vi "Tosca-Create Editor Event Registration.vi"(0 "FSM.Editor Ref":refnum<vi>, 5 "EventList Ref":refnum<vi>, 7 "Flags Ref":refnum<vi>, 9 "SigMan Ref":refnum<vi>) -> (4 "Event Registration Refnum":refnum<event-registration>)   [LabVIEW 2020]
uses:
  epl-vi-lib/Utility VIs/Controls/KListboxEx/KListboxEx.xctl
  FSM Graph VIs/LV Source/FSM Editor/FSM Editor.xctl
  epl-vi-lib/Utility VIs/Controls/KListboxEx/Events.ctl
  epl-vi-lib/Utility VIs/Controls/KListboxEx/Event Action.ctl
  epl-vi-lib/Utility VIs/Controls/KTable/KTable.xctl
  epl-vi-lib/Utility VIs/Controls/KTable/Events.ctl
  epl-vi-lib/Utility VIs/Controls/KTable/Event Data.ctl
  epl-vi-lib/Utility VIs/Controls/KTable/Event Type.ctl
  FSM Graph VIs/LV Source/FSM Editor/Events.ctl
  FSM Graph VIs/LV Source/FSM Editor/NodeAdded.ctl
  FSM Graph VIs/LV Source/FSM Editor/NodeSelected.ctl
  FSM Graph VIs/LV Source/FSM Editor/EdgeEventData.ctl
  epl-vi-lib/Signal Synthesis VIs/4th Generation/Controls/SignalManager/SignalManager.xctl
  epl-vi-lib/Signal Synthesis VIs/4th Generation/Controls/SignalManager/Events.ctl
  epl-vi-lib/Signal Synthesis VIs/4th Generation/Controls/SignalManager/Event Data.ctl
panel:
  out "SigMan":T1
  out "FSMEditor":T2
  out "Flags":T3
  out "EventList":T4
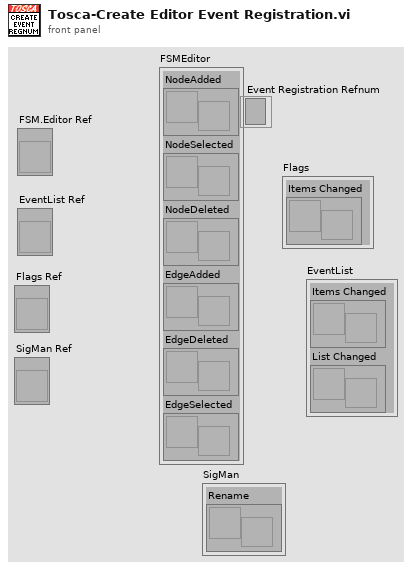
[diagram p1: front panel]
types:
  T1 = typedef "SignalManager.xctl/Events.ctl" = cluster{"Rename":refnum<user-event>}
  T2 = typedef "FSM Editor.xctl/Events.ctl" = cluster{"NodeAdded":refnum<user-event>, "NodeSelected":refnum<user-event>, "NodeDeleted":refnum<user-event>, "EdgeAdded":refnum<user-event>, "EdgeDeleted":refnum<user-event>, "EdgeSelected":refnum<user-event>}
  T3 = typedef "KTable.xctl/Events.ctl" = cluster{"Items Changed":refnum<user-event>}
  T4 = typedef "KListboxEx.xctl/Events.ctl" = cluster{"Items Changed":refnum<user-event>, "List Changed":refnum<user-event>}
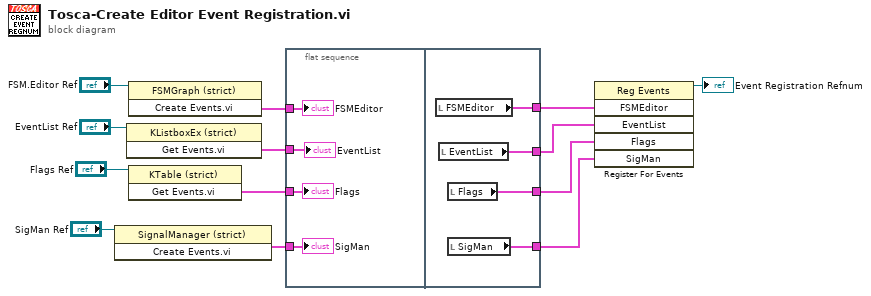
[diagram p0: block diagram]
diagram:
  n1 = invoke class="SignalManager (strict)" method="Create Events.vi"(reference="SigMan Ref") -> ("Create Events.vi"=w3:T1)  [unwired: 2 in, 2 out]
  n2 = invoke on="Invoke Node" class="KListboxEx (strict)" method="Get Events.vi"(reference="EventList Ref") -> ("Get Events.vi"=w10:T4)  [unwired: 2 in, 2 out]
  n3 = invoke on="Invoke Node" class="FSMGraph (strict)" method="Create Events.vi"(reference="FSM.Editor Ref") -> ("Create Events.vi"=w11:T2)  [unwired: 2 in, 2 out]
  n4 = invoke on="Invoke Node" class="KTable (strict)" method="Get Events.vi"(reference="Flags Ref") -> ("Get Events.vi"=w6:T3)  [unwired: 2 in, 2 out]
  n5 = flat-sequence {
    tunnel: w11 -> [w15]
    tunnel: w10 -> [w17]
    tunnel: w6 -> [w16]
    tunnel: w3 -> [w14]
    tunnel: [w21] -> w9
    tunnel: [w20] -> w8
    tunnel: [w19] -> w7
    tunnel: [w18] -> w2
    frame #0 {
      "EventList" <- w17
      "Flags" <- w16
      "FSMEditor" <- w15
      "SigMan" <- w14
    }
    frame #1 {
      n6 = local read "FSMEditor"() -> (w21:T2)
      n7 = local read "EventList"() -> (w20:T4)
      n8 = local read "Flags"() -> (w19:T3)
      n9 = local read "SigMan"() -> (w18:T1)
    }
  }
  n10 = register-events(w9, w8, w7, w2) -> (reference out=→"Event Registration Refnum":refnum<event-registration>)  [unwired: 2 in, 1 out]
